vi "Plot get newest and latest timestamp.vi"(11 "data history":T1) -> (0 "newest data":dbl, 1 "newest timestamp":u64, 2 "oldest timestamp":u64, 3 "data history":T1, 4 "Exists?":bool)   [LabVIEW 2021, in "RocketPlot.lvlib"]
uses:
  RocketPlot.lvlib
  TypeDefs/plot datapoint.ctl
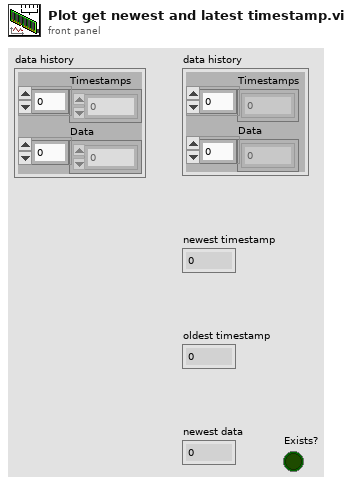
[diagram p1: front panel]
types:
  T1 = typedef "RocketPlot.lvlib/plot datapoint.ctl" = cluster{"Timestamps":u64[], "Data":dbl[]}
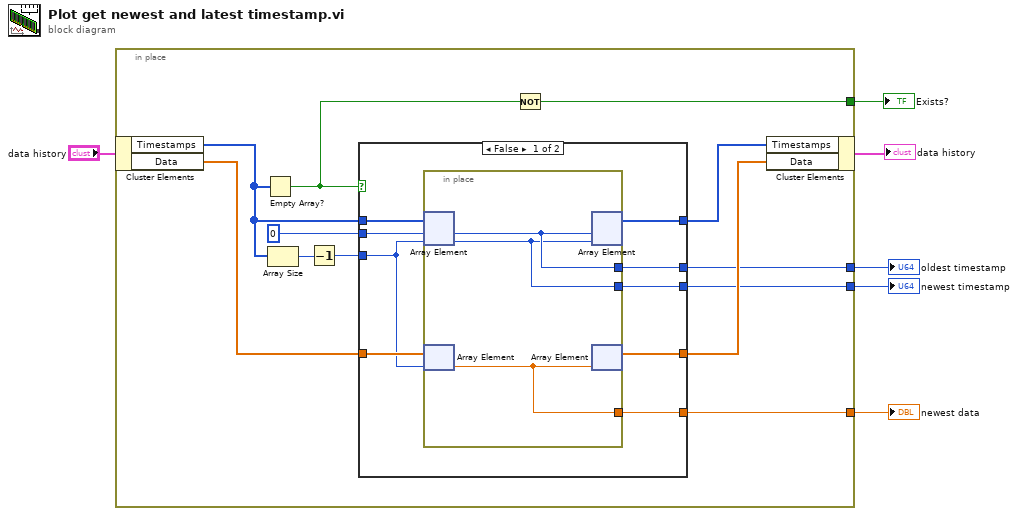
[diagram p0: block diagram]
diagram:
  n1 = in-place {
    in-place-border: [w11] -> w4
    in-place-border: [w10] -> w3
    in-place-border: [w9] -> w2
    in-place-border: [w7] -> w1
    n2 = in-place-cluster #1("data history") -> ("Timestamps"=w15:u64[], "Data"=w13:dbl[])
    n3 = Empty Array?(array=w15) -> (empty?=w8:bool)
    n4 = Array Size(array=w15) -> (size(s)=w18:i32)
    n5 = Decrement(x=w18) -> (x-1=w16:i32)
    n6 = case shown="False" w8 {
      tunnel: 0 -> [w23 _]
      tunnel: w16 -> [w19 _]
      tunnel: [w27 w32] -> w14
      tunnel: w15 -> [w26 w32]
      tunnel: w13 -> [w25 w31]
      tunnel: [w24 w31] -> w12
      tunnel: [w22 _] -> w11
      tunnel: [w21 _] -> w10
      tunnel: [w20 _] -> w9
      frame False {
        n7 = in-place {
          in-place-border: [w30] -> w22
          in-place-border: [w29] -> w21
          in-place-border: [w28] -> w20
          n8 = in-place-array #2(w26, w23, w19) -> (w30:u64, w29:u64)
          n9 = in-place-array #3(w25, w19) -> (w28:dbl)
          n10 = in-place-array #2(w30, w29) -> (w27:u64[])  [unwired: 2 out]
          n11 = in-place-array #3(w28) -> (w24:dbl[])  [unwired: 1 out]
        }
      }
      frame True {
      }
    }
    n12 = Not(x=w8) -> (.not. x?=w7:bool)
    n13 = in-place-cluster #1("Timestamps"=w14, "Data"=w12) -> (→"data history":T1)
  }
  "oldest timestamp" <- w4
  "newest timestamp" <- w3
  "newest data" <- w2
  "Exists?" <- w1
